vi "4 poprawione.vi"() -> ()   [LabVIEW 2013]
panel:
  out "2D Picture":picture
  out "Rescaled (x,y)":cluster{dbl, dbl}[](array[cluster])
  out "(X, X^2)":cluster{dbl, dbl}[](array[cluster])
  in  "N":dbl=250.0 format="%#_13g"
  out "A_W i A_H":cluster{dbl, dbl}
  out "r_W i r_H":cluster{dbl, dbl}
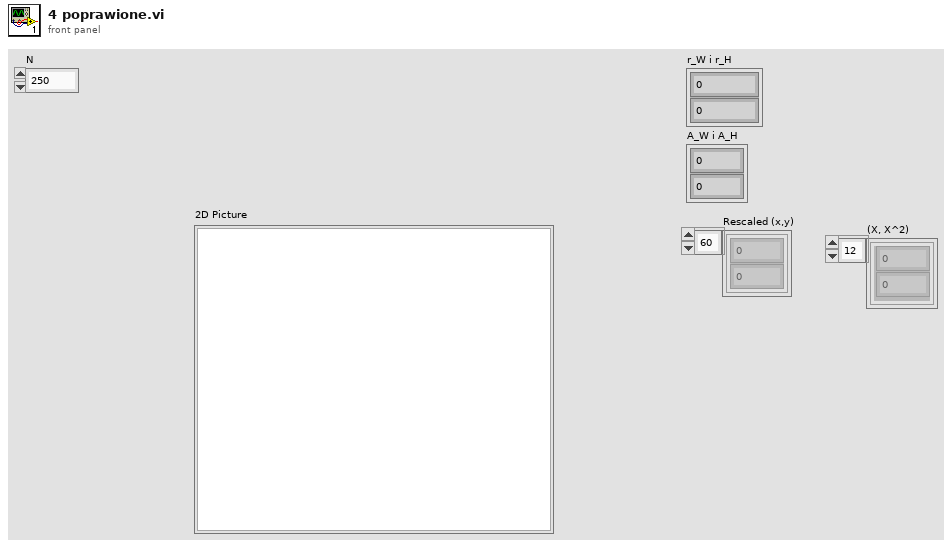
[diagram p1: front panel]
types:
  T1 = typedef "LVBoundsTypeDef.ctl" = cluster{"Width":u32, "Height":u32}
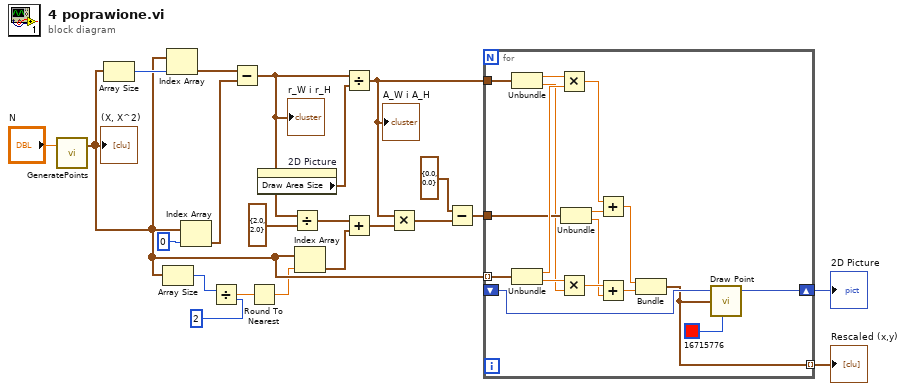
[diagram p0: block diagram]
diagram:
  n1 = call "GeneratePoints.vi"("N"="N") -> ("(X, X^2)"=w3:cluster{dbl, dbl}[])  [unwired: 1 in, 1 out]
  "(X, X^2)" <- w3
  n2 = Array Size(array=w3) -> (size(s)=w21:i32)
  n3 = Array Size(array=w3) -> (size(s)=w17:i32)
  n4 = Index Array(array=w3, index=w21) -> (element=w20:cluster{dbl, dbl})
  n5 = Index Array(array=w3, index=0) -> (element=w19:cluster{dbl, dbl})
  n6 = Divide(x=w17, y=2) -> (x/y=w2:dbl)
  n7 = Subtract(x=w20, y=w19) -> (x-y=w14:cluster{dbl, dbl})
  "r_W i r_H" <- w14
  n8 = Round To Nearest(number=w2) -> (nearest integer value=w1:dbl)
  n9 = property on="2D Picture" class="Pict"() -> ("Draw Area Size"=w4:T1)  [unwired: 2 in, 2 out]
  n10 = Divide(x=w14, y=cluster{dbl, dbl} {2.0, 2.0}) -> (x/y=w12:cluster{dbl, dbl})
  n11 = Index Array(array=w3, index=w1) -> (element=w15:cluster{dbl, dbl})
  n12 = Divide(x=w14, y=w4) -> (x/y=w9:cluster{dbl, dbl})
  "A_W i A_H" <- w9
  n13 = Add(x=w12, y=w15) -> (x+y=w11:cluster{dbl, dbl})
  n14 = Multiply(x=w9, y=w11) -> (x*y=w10:cluster{dbl, dbl})
  n15 = Subtract(x=cluster{dbl, dbl} {0.0, 0.0}, y=w10) -> (x-y=w8:cluster{dbl, dbl})
  n16 = for {
    tunnel: w3 -> [w39] mode=indexing
    tunnel: w9 -> [w36]
    tunnel: w8 -> [w35]
    shift-right: [w26] -> w5
    shift-left: _ -> [w25]
    tunnel: [w23] -> w6 mode=indexing
    n17 = Unbundle(w36) -> (w34:dbl, w31:dbl)
    n18 = Unbundle(w39) -> (w38:dbl, w32:dbl)
    n19 = Multiply(x=w34, y=w38) -> (x*y=w37:dbl)
    n20 = Multiply(x=w32, y=w31) -> (x*y=w30:dbl)
    n21 = Unbundle(w35) -> (w33:dbl, w29:dbl)
    n22 = Add(x=w37, y=w33) -> (x+y=w28:dbl)
    n23 = Add(x=w30, y=w29) -> (x+y=w27:dbl)
    n24 = Bundle(w28, w27) -> (w23:cluster{dbl, dbl})  [unwired: 1 in]
    n25 = call <vilib>:"Draw Point.vi"("picture"=w25, "point(x,y)"=w23, "color(black)"=u32 16715776) -> ("new picture"=w26:picture)  [unwired: 6 in]
  }
  "Rescaled (x,y)" <- w6
  "2D Picture" <- w5
